vi "SmoothRangeOfCoefficients.vi"(6 "LFSmoothingCeiling":dbl, 9 "LFSmoothingFloor":dbl, 10 "NyquistLimitedCoefficients In":dbl[](array[numeric]), 11 "Frequencies In":dbl[](array[numeric])) -> (0 "Coefficients Smoothed and Normalized":bool, 2 "SmoothingTerm":dbl format="%0.2f", 3 "NyquistLimitedCoefficients Out":dbl[](array[numeric]))   [LabVIEW 2012]
uses:
  <vilib>/Analysis/baseanly.llb/Mean (DBL).vi
  <vilib>/Analysis/NI_AALBase.lvlib
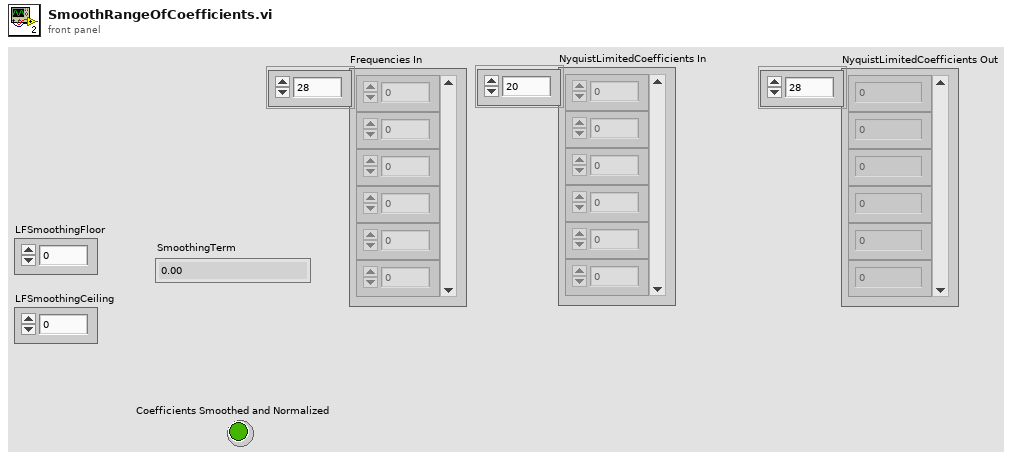
[diagram p1: front panel]
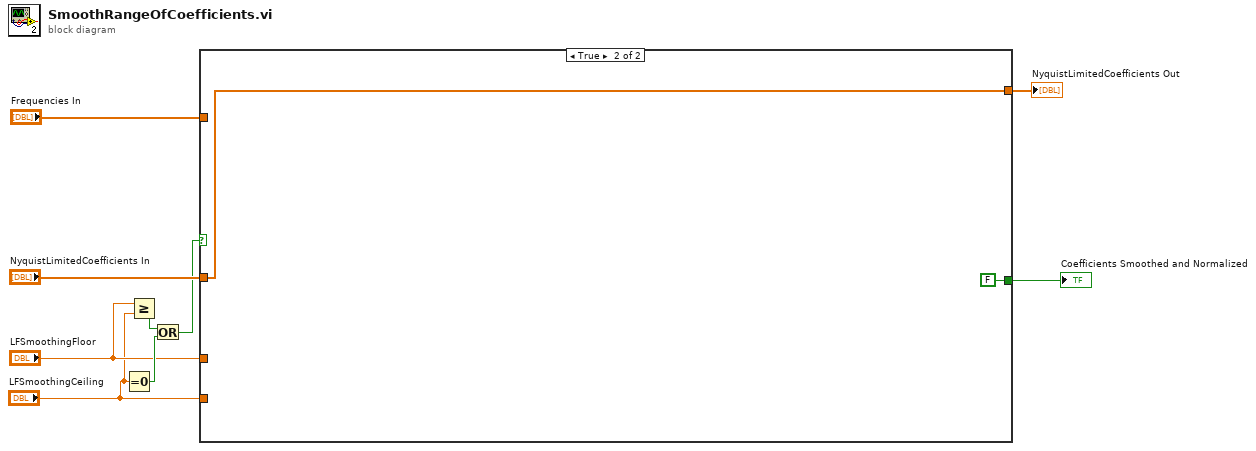
[diagram p0: block diagram]
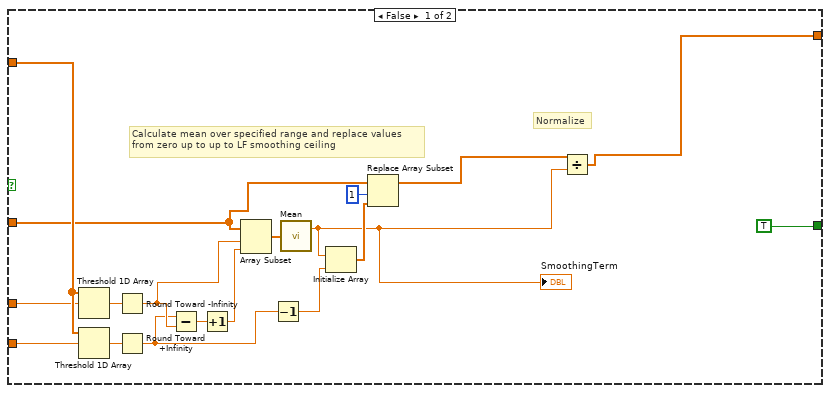
[diagram p2: hidden frame]
diagram:
  n1 = Equal To 0?(x="LFSmoothingCeiling") -> (x = 0?=w5:bool)
  n2 = Greater Or Equal?(x="LFSmoothingFloor", y="LFSmoothingCeiling") -> (x >= y?=w1:bool)
  n3 = Or(x=w1, y=w5) -> (x .or. y?=w4:bool)
  n4 = case shown="True" w4 {
    tunnel: "Frequencies In" -> [w26 _]
    tunnel: [w11 w29] -> w8
    tunnel: "NyquistLimitedCoefficients In" -> [w22 w29]
    tunnel: "LFSmoothingFloor" -> [w15 _]
    tunnel: "LFSmoothingCeiling" -> [w14 _]
    tunnel: [TRUE ("Coefficients Smoothed and Normalized") FALSE ("Coefficients Smoothed and Normalized")] -> w6
    frame False {
      # "Calculate mean over specified range and replace values\nfrom zero up to up to LF smoothing ceiling"
      # "Normalize"
      n5 = Threshold 1D Array(2:w15, 3:w26) -> (0:w18:dbl)  [unwired: 1 in]
      n6 = Threshold 1D Array(2:w14, 3:w26) -> (0:w19:dbl)  [unwired: 1 in]
      n7 = Round Toward -Infinity(1:w18) -> (0:w23:dbl)
      n8 = Round Toward +Infinity(x=w19) -> (ceil(x): smallest int >= x=w17:dbl)
      n9 = Subtract(x=w17, y=w23) -> (x-y=w20:dbl)
      n10 = Increment(x=w20) -> (x+1=w25:dbl)
      n11 = Array Subset(array=w22, index=w23, length=w25) -> (w21:dbl[])
      n12 = Decrement(x=w17) -> (x-1=w16:dbl)
      n13 = call-poly <vilib>:"Mean.vi"("X"=w21) -> ("mean"=w13:dbl)  [unwired: 1 out]
      "SmoothingTerm" <- w13
      n14 = Initialize Array(w13, w16) -> (w24:dbl[])
      n15 = Replace Array Subset(array=w22, new element=w24, index=1) -> (w12:dbl[])
      n16 = Divide(x=w12, y=w13) -> (x/y=w11:dbl[])
    }
    frame True {
    }
  }
  "NyquistLimitedCoefficients Out" <- w8
  "Coefficients Smoothed and Normalized" <- w6
